vi "1.vi"() -> ()   [LabVIEW 2016]
uses:
  <vilib>/addons/Time Frequency Analysis/Spectrogram.llb/TFA Fast Gabor Spectrogram (Waveform).vi
  <vilib>/addons/Time Frequency Analysis/_control.llb/TFA Configure Spectrogram Indicator (Predefined Color Table).vi
  <vilib>/Analysis/NI_AALPro.lvlib
  <vilib>/addons/_Advanced Signal Processing/NI_AdvSigProcTFA.lvlib
panel:
  out "Original signal 2":dynamicdata(graph)
  out "Averaged_filtered_Hilbert":waveform(dbl)(graph)
  out "Spectrogram of Gabor":dbl[][](graph)
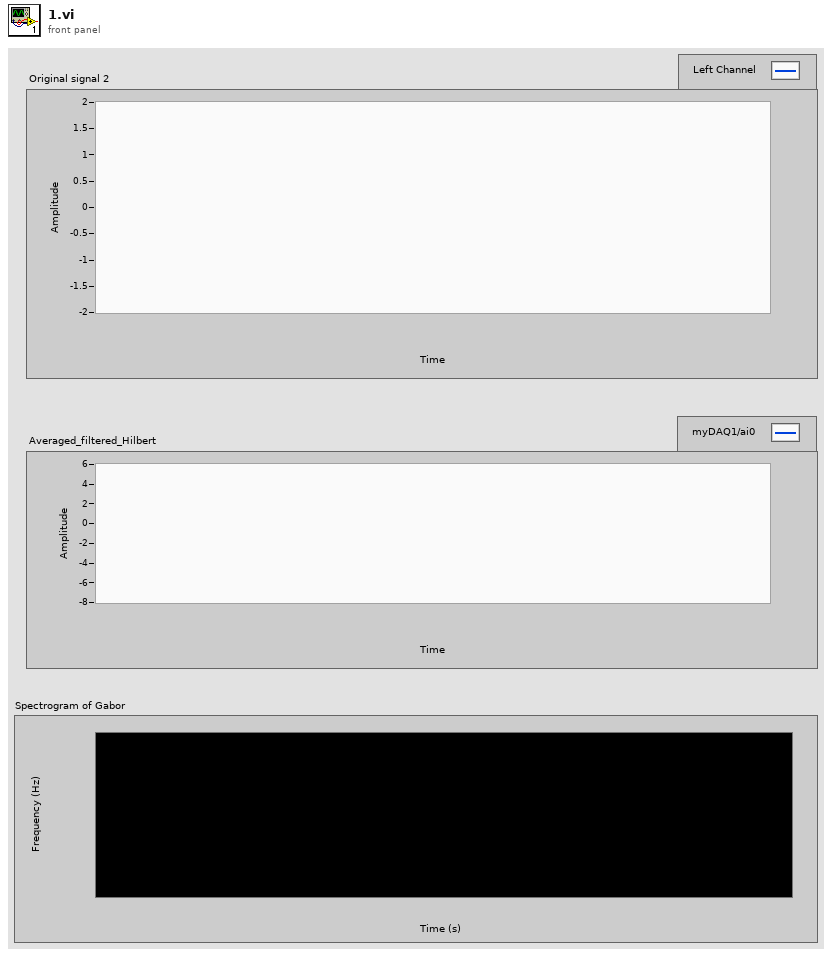
[diagram p1: front panel]
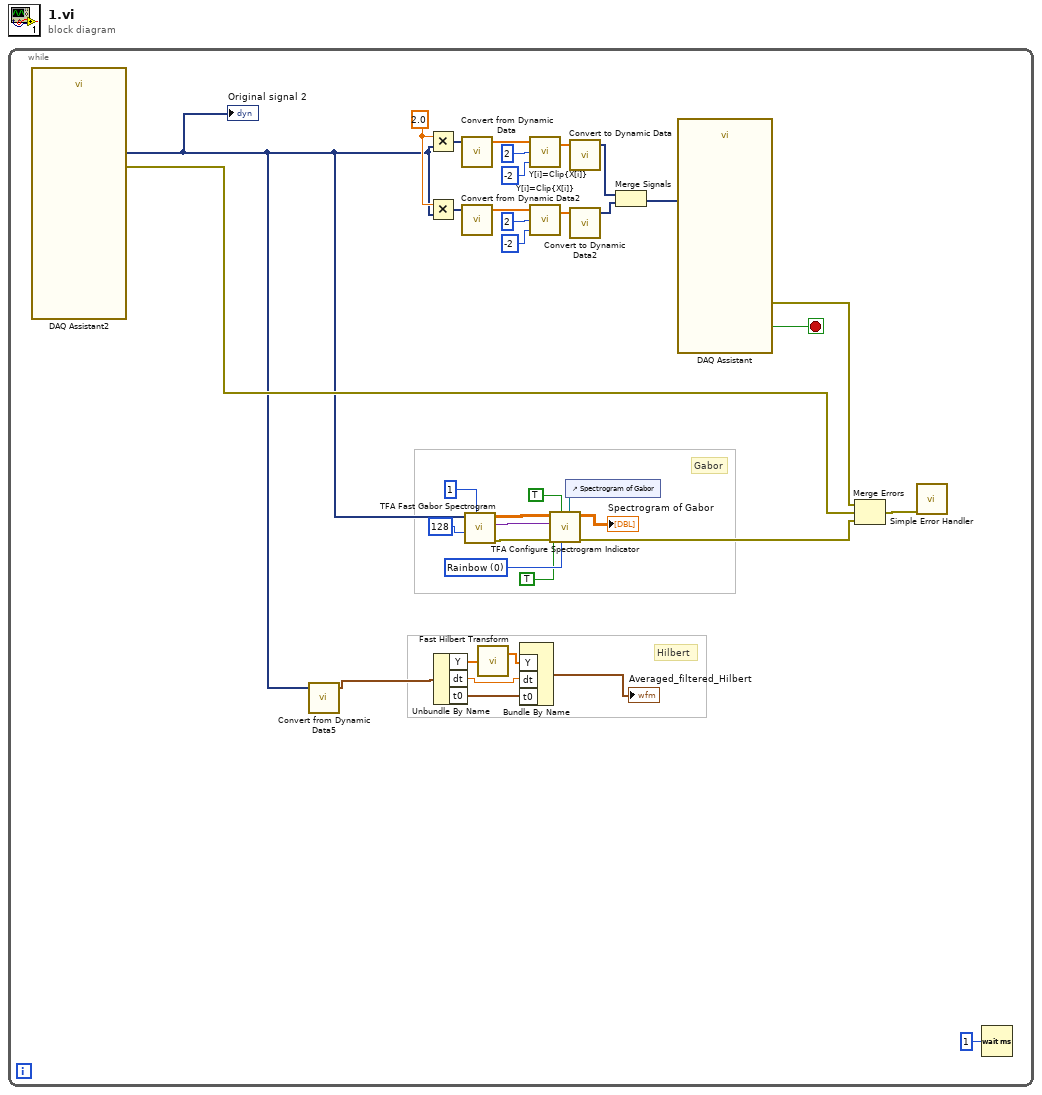
[diagram p0: block diagram]
diagram:
  n1 = while {
    stop <- w23 stop-if-true
    w15 = u16 0 items=["Rainbow", "Inverse gray", "Gray"] ("color table")
    w37 = 2.0
    # "Hilbert"
    # "Gabor"
    n2 = call "DAQ Assistant2"() -> ("data"=w2:dynamicdata, "error out"=w12:errorcluster)  [unwired: 16 in, 2 out]
    "Original signal 2" <- w2
    n3 = call "Convert from Dynamic Data5"("Dynamic Data Type"=w2) -> ("Waveform"=w4:waveform(dbl))  [unwired: 3 in]
    n4 = Multiply(x=w37, y=w2) -> (x*y=w34:dynamicdata)
    n5 = Multiply(x=w37, y=w2) -> (x*y=w28:dynamicdata)
    n6 = Unbundle By Name(w4) -> ("Y"=w8:dbl[], "dt"=w6:dbl, "t0"=w5:timestamp)
    n7 = call "Convert from Dynamic Data"("Dynamic Data Type"=w34) -> ("Array"=w33:dbl[])  [unwired: 3 in]
    n8 = call "Convert from Dynamic Data2"("Dynamic Data Type"=w28) -> ("Array"=w27:dbl[])  [unwired: 3 in]
    n9 = call-poly <vilib>:"TFA Fast Gabor Spectrogram.vi"("order"=1, "Gaussian window length"=128, "signal"=w2) -> ("error out"=w16:errorcluster, "scale info"=w21:variant, "spectrogram"=w22:dbl[][])  [unwired: 2 in, 4 out]
    n10 = call <vilib>:"Fast Hilbert Transform.vi"("X"=w8) -> ("Hilbert{X}"=w7:dbl[])  [unwired: 1 out]
    n11 = Bundle By Name("Y"=w7, "dt"=w6, "t0"=w5) -> (→"Averaged_filtered_Hilbert":waveform(dbl))  [unwired: 1 in]
    n12 = call <vilib>:"Y[i]=Clip{X[i]}.vi"("lower limit"=-2, "upper limit"=2, "Input Array"=w33) -> ("Clipped Array"=w32:dbl[])  [unwired: 1 out]
    n13 = call <vilib>:"Y[i]=Clip{X[i]}.vi"("lower limit"=-2, "upper limit"=2, "Input Array"=w27) -> ("Clipped Array"=w26:dbl[])  [unwired: 1 out]
    n14 = control-ref of="Spectrogram of Gabor"() -> (w19:refnum<vi>)
    n15 = call-poly <vilib>:"TFA Configure Spectrogram Indicator.vi"("reference of TF spectrogram indicator"=w19, "color table"=w15, "dB on? (F)"=TRUE ("dB"), "error in (no error)"=w16, "ignore timestamp? (F)"=TRUE, "scale info"=w21, "spectrogram"=w22) -> ("error out"=w10:errorcluster, "TF spectrogram indicator"=→"Spectrogram of Gabor":dbl[][])  [unwired: 3 out]
    n16 = call "Convert to Dynamic Data"("Array"=w32) -> ("Dynamic Data Type"=w31:dynamicdata)  [unwired: 3 in]
    n17 = call "Convert to Dynamic Data2"("Array"=w26) -> ("Dynamic Data Type"=w25:dynamicdata)  [unwired: 3 in]
    n18 = Merge Signals(w31, w25) -> (w24:dynamicdata)
    n19 = call "DAQ Assistant"("data"=w24) -> ("stopped"=w23:bool, "error out"=w11:errorcluster)  [unwired: 16 in, 1 out]
    n20 = Merge Errors(w11, w12, w10) -> (w13:errorcluster)
    n21 = call <vilib>:"Simple Error Handler.vi"("error in (no error)"=w13) -> ()  [unwired: 1 in, 8 out]
    n22 = Wait (ms)(milliseconds to wait=u32 1) -> ()  [unwired: 1 out]
  }
